vi "Get Path Regex.vi"(8 "error in (no error)":errorcluster, 11 "Registration in":refnum<class "Registration.lvclass">) -> (0 "error out":errorcluster, 2 "Path Regex":string, 3 "Registration out":refnum<class "Registration.lvclass">)   [LabVIEW 2020, in "Summer of LabVIEW.lvlib" / "Registration.lvclass"]
uses:
  Registration.lvclass
  Registration.lvclass/Registration.ctl
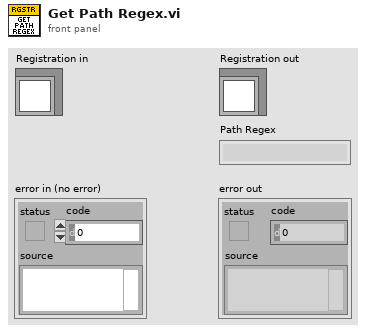
[diagram p1: front panel]
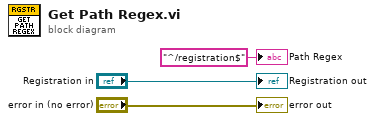
[diagram p0: block diagram]
diagram:
  "error out" <- "error in (no error)"
  "Registration out" <- "Registration in"
  "Path Regex" <- "^/registration$" ("Path Regex")
